vi "start.vi"(8 "error in (no error)":errorcluster, 10 "ILCConfig":T1 {"ADC PGA Gain" max=7}, 11 "ILC in":refnum<class "ILC.lvclass">) -> (0 "error out":errorcluster, 2 "configString":string, 3 "ILC out":refnum<class "ILC.lvclass">)   [LabVIEW 2013, in "ILCCommon.lvlib" / "ILC.lvclass"]
uses:
  <userlib>/Common/ILC/ILC/ILC.lvclass
  <userlib>/Common/ILC/Configuration/ILCConfig.ctl
  <userlib>/Common/ILC/Configuration/InputChannels.ctl
  <userlib>/Common/ILC/Configuration/ScanRate_Hz_MultichannelOptions.ctl
  <userlib>/Common/ILC/Configuration/ILCConfiguration.lvlib
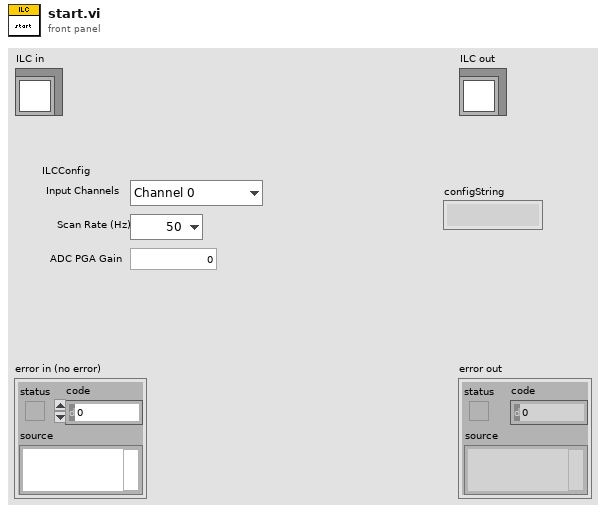
[diagram p1: front panel]
types:
  T1 = typedef "ILCCommon.lvlib/ILCConfiguration.lvlib/ILCConfig.ctl" = cluster{"Input Channels":T2, "Scan Rate (Hz) ":T3, "ADC PGA Gain":u8}
  T2 = typedef "ILCCommon.lvlib/ILCConfiguration.lvlib/InputChannels.ctl" = enum16{"Channel 0", "3 Channels", "5 Channels"}
  T3 = typedef "ILCCommon.lvlib/ILCConfiguration.lvlib/ScanRate_Hz_MultichannelOptions.ctl" = enum16{"50", "60", "100", "120", "200", "240", "300", "400", "480", "600", "1200", "2400", "4800"}
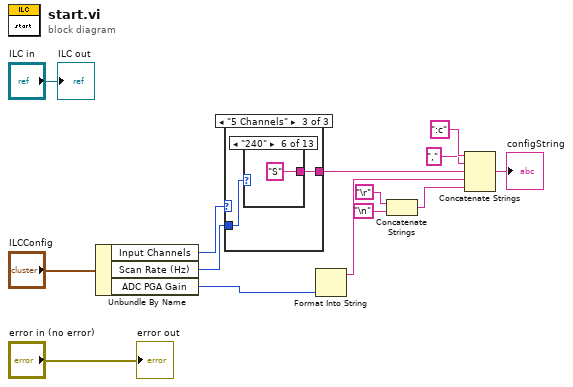
[diagram p0: block diagram]
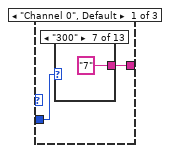
[diagram p2: hidden frame]
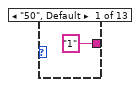
[diagram p3: hidden frame]
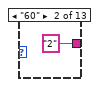
[diagram p4: hidden frame]
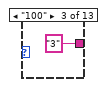
[diagram p5: hidden frame]
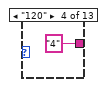
[diagram p6: hidden frame]
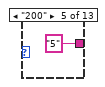
[diagram p7: hidden frame]
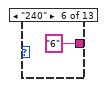
[diagram p8: hidden frame]
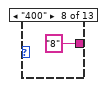
[diagram p9: hidden frame]
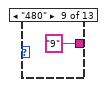
[diagram p10: hidden frame]
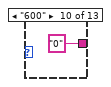
[diagram p11: hidden frame]
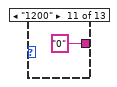
[diagram p12: hidden frame]
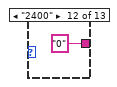
[diagram p13: hidden frame]
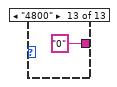
[diagram p14: hidden frame]
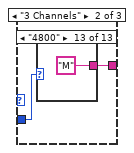
[diagram p15: hidden frame]
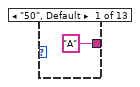
[diagram p16: hidden frame]
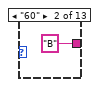
[diagram p17: hidden frame]
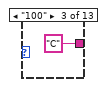
[diagram p18: hidden frame]
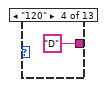
[diagram p19: hidden frame]
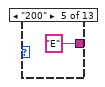
[diagram p20: hidden frame]
diagram:
  n1 = Unbundle By Name("ILCConfig") -> ("Input Channels"=w7:T2, "Scan Rate (Hz)"=w6:T3, "ADC PGA Gain"=w3:u8)
  n2 = case shown="\"5 Channels\"" w7 {
    tunnel: w6 -> [w16 w31 w46]
    tunnel: [w15 w30 w45] -> w5
    frame "Channel 0", Default {
      n3 = case shown="\"300\"" w16 {
        tunnel: ["1" ("string") "2" ("string") "3" ("string") "4" ("string") "5" ("string") "6" ("string") "7" ("string") "8" ("string") "9" ("string") "0" ("string") "0" ("string") "0" ("string") "0" ("string")] -> w15
        frame "50", Default {
        }
        frame "60" {
        }
        frame "100" {
        }
        frame "120" {
        }
        frame "200" {
        }
        frame "240" {
        }
        frame "300" {
        }
        frame "400" {
        }
        frame "480" {
        }
        frame "600" {
        }
        frame "1200" {
        }
        frame "2400" {
        }
        frame "4800" {
        }
      }
    }
    frame "3 Channels" {
      n4 = case shown="\"4800\"" w31 {
        tunnel: ["A" ("string") "B" ("string") "C" ("string") "D" ("string") "E" ("string") "F" ("string") "G" ("string") "H" ("string") "I" ("string") "J" ("string") "K" ("string") "L" ("string") "M" ("string")] -> w30
        frame "50", Default {
        }
        frame "60" {
        }
        frame "100" {
        }
        frame "120" {
        }
        frame "200" {
        }
        frame "240" {
        }
        frame "300" {
        }
        frame "400" {
        }
        frame "480" {
        }
        frame "600" {
        }
        frame "1200" {
        }
        frame "2400" {
        }
        frame "4800" {
        }
      }
    }
    frame "5 Channels" {
      n5 = case shown="\"240\"" w46 {
        tunnel: ["N" ("string") "O" ("string") "P" ("string") "Q" ("string") "R" ("string") "S" ("string") "T" ("string") "U" ("string") "V" ("string") "W" ("string") "X" ("string") "Y" ("string") "Z" ("string")] -> w45
        frame "50", Default {
        }
        frame "60" {
        }
        frame "100" {
        }
        frame "120" {
        }
        frame "200" {
        }
        frame "240" {
        }
        frame "300" {
        }
        frame "400" {
        }
        frame "480" {
        }
        frame "600" {
        }
        frame "1200" {
        }
        frame "2400" {
        }
        frame "4800" {
        }
      }
    }
  }
  n6 = Format Into String(w3) -> (resulting string=w2:string)  [unwired: 3 in, 1 out]
  n7 = Concatenate Strings("\r", "\n") -> (w4:string)
  n8 = Concatenate Strings(":c" ("string"), "," ("string"), w5, w2, w4) -> (→"configString":string)
  "error out" <- "error in (no error)"
  "ILC out" <- "ILC in"
